vi "SubPanel_Oscilloscope_Block_Rev11_v2.vi"(2 "error input":errorcluster, 3 "Oscilloscope Configuration Input Array":T2(array[cluster]) {"vertical coupling" items=["AC", "DC", "Ground"]}) -> (0 "error out":errorcluster, 1 "Oscilloscope Configuration Output Array":T2(array[cluster]) {"vertical coupling" items=["AC", "DC", "Ground"]})   [LabVIEW 2019]
uses:
  Controls/OscilloscopeBlockControl.ctl
  <instrlib>/niScope/Controls/niScope vertical coupling.ctl
  <instrlib>/niScope/Configure/Trigger/niScope Configure Trigger Software.vi
panel:
  out "Oscilloscope Configuration Array Indicator":T2(array[cluster]) {"vertical coupling" items=["AC", "DC", "Ground"]}
  in  "Remove An Oscilloscope":bool
  in  "Oscilloscope Configuration Input Array":T3(array[cluster]) {"vertical coupling" items=["AC", "DC", "Ground"]}
  out "Horizontal:Actual Record Length":i32
  out "Configuration Errors":errorcluster
  in  "Oscilloscope Block Parameters":T4={"Oscilloscope"="", "channel names list"="", "vertical range"=10.0, "vertical coupling"=1, "Channel 0 50 ohms?"=FALSE, "50 ohm vertical range (V)"=10.0, "min record length"=1000, "min sample rate"=20000000.0} {"min sample rate" format="%^.2e"; "vertical coupling" items=["AC", "DC", "Ground"]}
  in  "EXIT SubVI":bool
  in  "Apply Configuration":bool
  # "Instructions\n\nSelect Oscilloscope Resource under \"Oscilloscope\"\n\nin a comma separate form (line 1, line 2, ...) type in the channel names of the device. \nIMPORTANT NOTE: \"line 1, line 2, ...\" will correspond to \"channel 0, channel 1, ...\" for each oscilloscope resource\n\nset the vertical range (no greater than 30)\n\nset the vertical coupling (dc) \n\nSet the channel 0 to 50 ohm impedance if you have something that requires 50 ohms to measure\n\nset 50 ohm vertical range if you have selected channel 0 50 ohms as true (ensure that it is no greater than 10\n\nmin record length (1000)\n\nmin sample rate (20e6) if you want a higher resolution, you increase the sample rate\n\npress apply configuration \n\nreview the instrument array above echoing your parameters created\n\nif you wish to remove a resource, select the oscilloscope resource in the \"oscillscope\" drop down\n\npress \"remove an oscilloscope\"\n\nonce fully configured, press \"EXIT\""
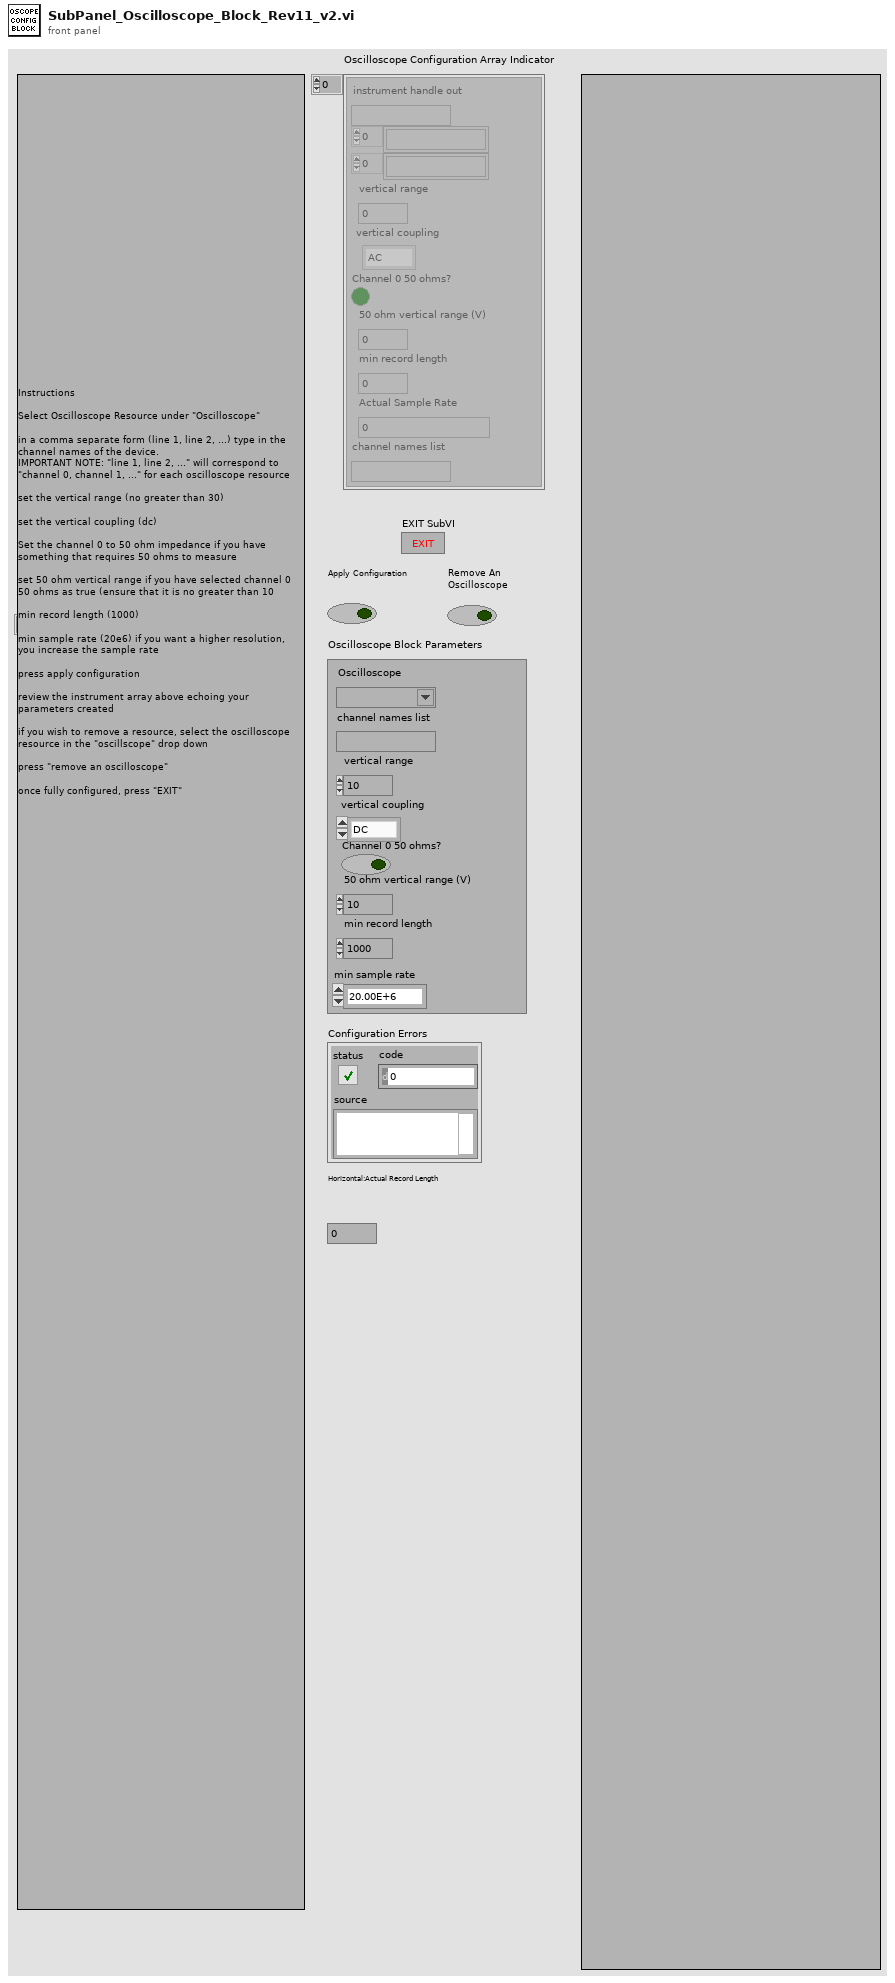
[diagram p1: front panel]
types:
  T1 = typedef "niScope vertical coupling.ctl" = i32
  T2 = cluster{"instrument handle out":refnum<k15>, string[], string[], "vertical range":dbl, "vertical coupling":T1, "Channel 0 50 ohms?":bool, "50 ohm vertical range (V)":dbl, "min record length":i32, "Actual Sample Rate":dbl, "channel names list":string}[]
  T3 = cluster{"instrument handle out":refnum<k15>, "channel numbers array":string[], "channel names array":string[], "vertical range":dbl, "vertical coupling":T1, "Channel 0 50 ohms?":bool, "50 ohm vertical range (V)":dbl, "min record length":i32, "Actual Sample Rate":dbl}[]
  T4 = typedef "OscilloscopeBlockControl.ctl" = cluster{"Oscilloscope":refnum<k15>, "channel names list":string, "vertical range":dbl, "vertical coupling":T1, "Channel 0 50 ohms?":bool, "50 ohm vertical range (V)":dbl, "min record length":i32, "min sample rate":dbl}
  T5 = cluster{"instrument handle out":refnum<k15>, string[], string[], "vertical range":dbl, "vertical coupling":T1, "Channel 0 50 ohms?":bool, "50 ohm vertical range (V)":dbl, "min record length":i32, "Actual Sample Rate":dbl, string}
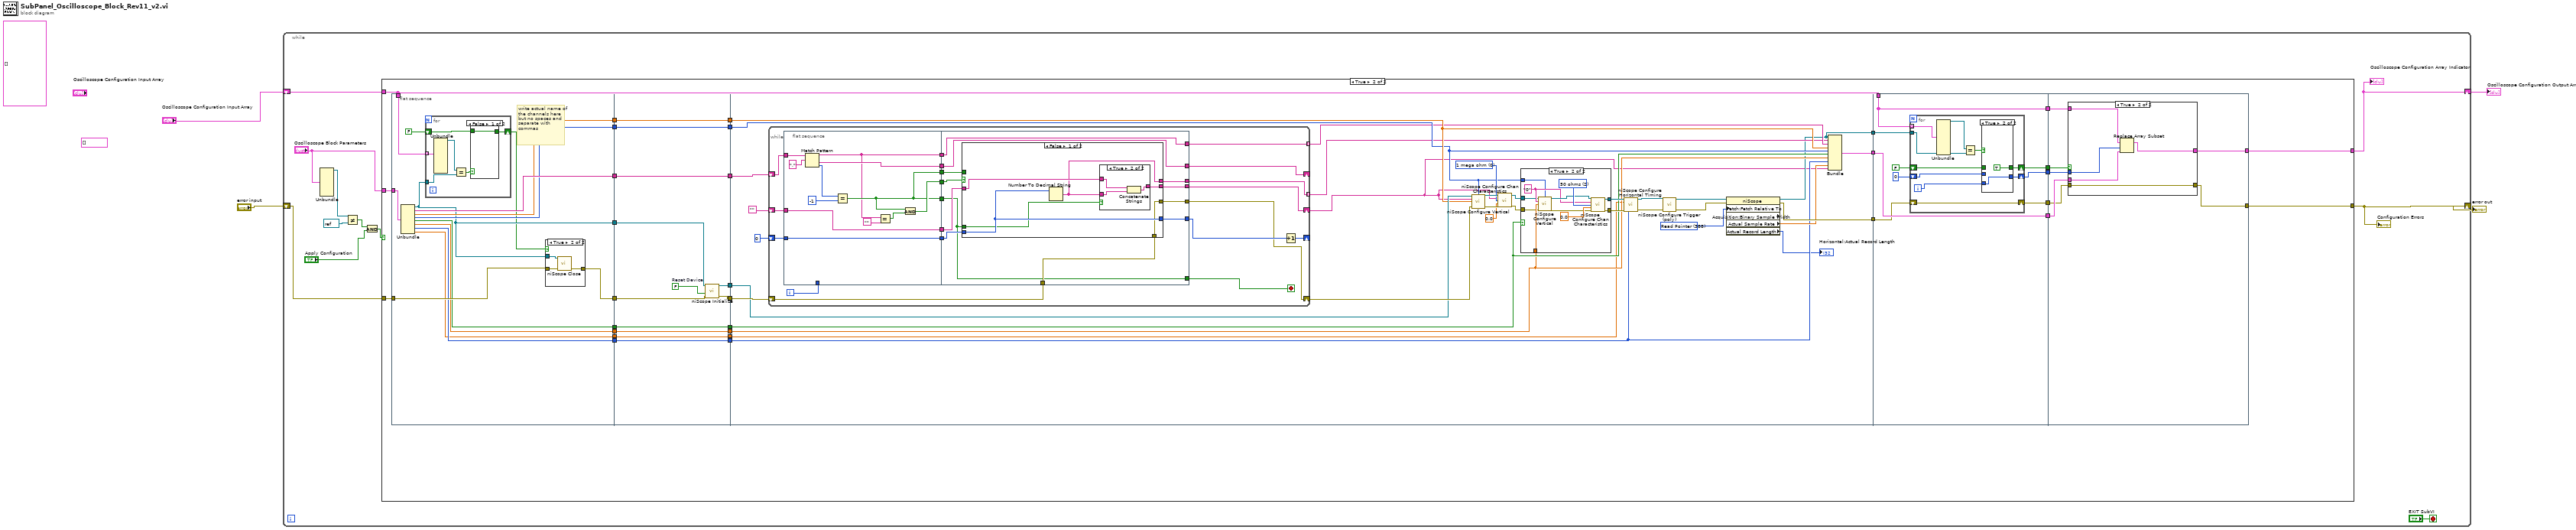
[diagram p0: block diagram]
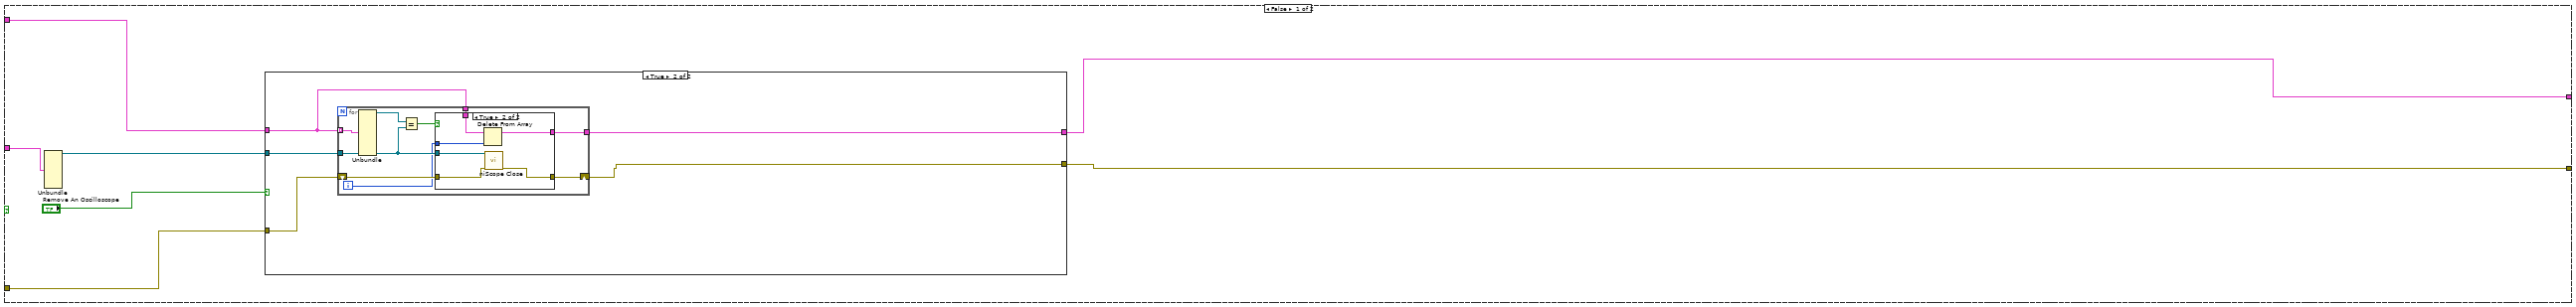
[diagram p2: hidden frame]
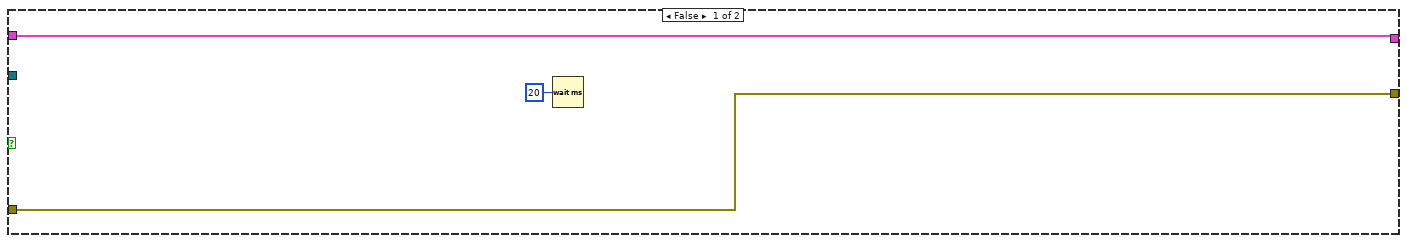
[diagram p3: hidden frame]
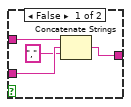
[diagram p7: hidden frame]
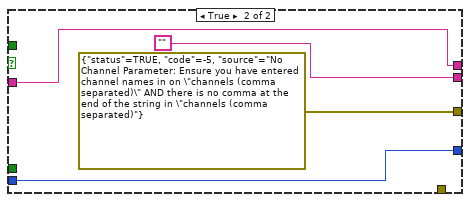
[diagram p8: hidden frame]
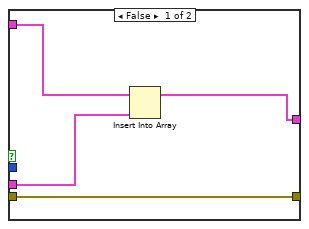
[diagram p11: hidden frame]
diagram:
  (unwired) T2 []
  (unwired) T3 [] ("Oscilloscope Configuration Input Array")
  n1 = while {
    shift-right: [w15] -> w4
    shift-left: "error input" -> [w13]
    shift-right: [w5] -> w1
    shift-left: "Oscilloscope Configuration Input Array" -> [w12]
    stop <- "EXIT SubVI" stop-if-true
    n2 = Unbundle("Oscilloscope Block Parameters") -> ("Oscilloscope"=w9:refnum<k15>)  [unwired: 7 out]
    n3 = Not Equal?(x=w9, y=refnum<k15> refnum ("resource name")) -> (x != y?=w8:bool)
    n4 = And(x=w8, y="Apply Configuration") -> (x .and. y?=w6:bool)
    n5 = case shown="True" w6 {
      tunnel: w13 -> [w19 w78]
      tunnel: [w18 w73] -> w15
      tunnel: [w16 w72] -> w5
      tunnel: w12 -> [w17 w48]
      tunnel: "Oscilloscope Block Parameters" -> [w22 w49]
      frame False {
        n6 = Unbundle(w22) -> ("Oscilloscope"=w20:refnum<k15>)  [unwired: 7 out]
        n7 = case shown="True" "Remove An Oscilloscope" {
          tunnel: w20 -> [_ w30]
          tunnel: w19 -> [w25 w29]
          tunnel: [w25 w26] -> w18
          tunnel: w17 -> [w23 w28]
          tunnel: [w23 w27] -> w16
          frame False {
            n8 = Wait (ms)(milliseconds to wait=u32 20) -> ()  [unwired: 1 out]
          }
          frame True {
            n9 = for {
              tunnel: w28 -> [w39] mode=indexing
              tunnel: w30 -> [w36]
              shift-right: [w34] -> w26
              shift-left: w29 -> [w35]
              tunnel: w28 -> [w33]
              tunnel: [w31] -> w27
              i -> [w32]
              n10 = Unbundle(w39) -> ("instrument handle out"=w38:refnum<k15>)  [unwired: 9 out]
              n11 = Equal?(x=w38, y=w36) -> (x = y?=w37:bool)
              n12 = case shown="True" w37 {
                tunnel: w36 -> [_ w47]
                tunnel: w35 -> [w41 w46]
                tunnel: [w41 w45] -> w34
                tunnel: w33 -> [w40 w44]
                tunnel: w32 -> [_ w43]
                tunnel: [w40 w42] -> w31
                frame False {
                }
                frame True {
                  n13 = Delete From Array(array=w44, index=w43) -> (array with subset deleted=w42:T2)  [unwired: 1 in, 1 out]
                  n14 = call <instrlib>:"niScope Close.vi"("instrument handle"=w47, "error in"=w46) -> ("error out"=w45:errorcluster)  [unwired: 13 in]
                }
              }
            }
          }
        }
      }
      frame True {
        n15 = flat-sequence {
          tunnel: w78 -> [w92]
          tunnel: [w91] -> w74
          tunnel: [w81] -> w71
          tunnel: [w90] -> w70
          tunnel: [w89] -> w68
          tunnel: [w88] -> w66
          tunnel: [w87] -> w64
          tunnel: [w86] -> w62
          tunnel: [w85] -> w60
          tunnel: [w84] -> w58
          tunnel: w49 -> [w83]
          tunnel: w48 -> [w82]
          tunnel: [w112] -> w77
          tunnel: [w114] -> w76
          tunnel: [w113] -> w75
          tunnel: w74 -> [w115]
          tunnel: w71 -> [w111]
          tunnel: w70 -> [w112]
          tunnel: [w110] -> w69
          tunnel: w68 -> [w110]
          tunnel: [w109] -> w67
          tunnel: w66 -> [w109]
          tunnel: [w108] -> w65
          tunnel: w64 -> [w108]
          tunnel: [w107] -> w63
          tunnel: w62 -> [w107]
          tunnel: [w106] -> w61
          tunnel: w60 -> [w106]
          tunnel: [w105] -> w59
          tunnel: w58 -> [w105]
          tunnel: w75 -> [w131]
          tunnel: w76 -> [w134]
          tunnel: w77 -> [w120]
          tunnel: w69 -> [w130]
          tunnel: w67 -> [w129]
          tunnel: w65 -> [w128]
          tunnel: w63 -> [w127]
          tunnel: w61 -> [w126]
          tunnel: w59 -> [w125]
          tunnel: [w137] -> w57
          tunnel: [w132] -> w56
          tunnel: [w121] -> w55
          tunnel: w57 -> [w225]
          tunnel: w56 -> [w232]
          tunnel: w55 -> [w231]
          tunnel: w48 -> [w227]
          tunnel: [w224] -> w54
          tunnel: [w232] -> w53
          tunnel: [w228] -> w52
          tunnel: [w227] -> w51
          tunnel: [w226] -> w50
          tunnel: [w250] -> w72
          tunnel: [w247] -> w73
          tunnel: w54 -> [w248]
          tunnel: w53 -> [w249]
          tunnel: w52 -> [w253]
          tunnel: w51 -> [w252]
          tunnel: w50 -> [w251]
          frame #0 {
            # "write actual name of the channels here but no spaces and separate with commas"
            n16 = Unbundle(w83) -> ("Oscilloscope"=w81:refnum<k15>, "channel names list"=w90:string, "vertical range"=w89:dbl, "vertical coupling"=w88:T1, "Channel 0 50 ohms?"=w87:bool, "50 ohm vertical range (V)"=w86:dbl, "min record length"=w85:i32, "min sample rate"=w84:dbl)
            n17 = for {
              tunnel: w82 -> [w98] mode=indexing
              tunnel: w81 -> [w97]
              shift-right: [w94] -> w79
              shift-left: FALSE -> [w93]
              n18 = Unbundle(w98) -> ("instrument handle out"=w96:refnum<k15>)  [unwired: 9 out]
              n19 = Equal?(x=w96, y=w97) -> (x = y?=w95:bool)
              n20 = case shown="False" w95 {
                selector: w95 -> [_ w100]
                tunnel: [w99 w100] -> w94
                tunnel: w93 -> [w99 _]
                frame False {
                }
                frame True {
                }
              }
            }
            n21 = case shown="True" w79 {
              tunnel: w81 -> [_ w102]
              tunnel: w92 -> [w101 w104]
              tunnel: [w101 w103] -> w91
              frame False {
              }
              frame True {
                n22 = call <instrlib>:"niScope Close.vi"("instrument handle"=w102, "error in"=w104) -> ("error out"=w103:errorcluster)  [unwired: 13 in]
              }
            }
          }
          frame #1 {
            w116 = FALSE  # Reset Device
            n23 = call <instrlib>:"niScope Initialize.vi"("resource name"=w111, "reset device"=w116, "error in"=w115) -> ("instrument handle"=w113:refnum<k15>, "error out"=w114:errorcluster)  [unwired: 11 in]
          }
          frame #2 {
            w140 = 388 items=["Start"=482, "Trigger"=483, "Pretrigger"=477, "Now"=481, "Read Pointer"=388] ("Fetch:Fetch Relative To")
            w146 = u32 0 items=["1 mega ohm"=0, "50 ohms"=2] ("input impedance")
            n24 = while {
              shift-right: [w168] -> _
              shift-left: w120 -> [w169]
              shift-right: [w156] -> _
              shift-left: 0 -> [w161]
              shift-right: [w153] -> w119
              shift-left: "" -> [w159]
              tunnel: [w152] -> w124 mode=indexing
              shift-right: [w154] -> w149
              shift-left: w134 -> [w158]
              tunnel: [w150] -> w123 mode=indexing
              i -> [w167]
              stop <- w166 stop-if-true
              n25 = flat-sequence {
                tunnel: w169 -> [w179]
                tunnel: w167 -> [_]
                tunnel: [w177] -> w165
                tunnel: [w171] -> w164
                tunnel: [w172] -> w163
                tunnel: [w176] -> w162
                tunnel: w161 -> [w176]
                tunnel: [w175] -> w160
                tunnel: w159 -> [w175]
                tunnel: [w171] -> w155
                tunnel: [w170] -> w151
                tunnel: w165 -> [w193]
                tunnel: w164 -> [w184]
                tunnel: w163 -> [w192]
                tunnel: w162 -> [w190]
                tunnel: w160 -> [w189]
                tunnel: w158 -> [w188]
                tunnel: [w193] -> w168
                tunnel: [w184] -> w166
                tunnel: [w191] -> w153
                tunnel: [w187] -> w154
                tunnel: [w186] -> w157
                tunnel: w155 -> [w185]
                tunnel: [w183] -> w152
                tunnel: w151 -> [w183]
                tunnel: [w182] -> w150
                frame #0 {
                  n26 = Match Pattern(string=w179, regular expression=",") -> (before substring=w170:string, after substring=w177:string, offset past match=w181:i32)  [unwired: 1 in, 1 out]
                  n27 = Equal?(x=w181, y=-1) -> (x = y?=w171:bool)
                  n28 = Equal?(x=w170, y="") -> (x = y?=w173:bool)
                  n29 = And(x=w171, y=w173) -> (x .and. y?=w172:bool)
                }
                frame #1 {
                  n30 = case shown="False" w192 {
                    tunnel: [w195 ""] -> w191
                    tunnel: w190 -> [w199 w209]
                    tunnel: w189 -> [w197 w207]
                    tunnel: [w199 w209] -> w186
                    tunnel: w188 -> [w198 _]
                    tunnel: [w198 errorcluster {"status"=TRUE, "code"=-5, "source"="No Channel Parameter: Ensure you have entered channel names in on \"channels (comma separated)\" AND there is no comma at the end of the string in \"channels (comma separated)"} ("error out")] -> w187
                    tunnel: w185 -> [_ _]
                    tunnel: w184 -> [w196 _]
                    tunnel: [w194 w207] -> w182
                    frame False {
                      n31 = Number To Decimal String(number=w199) -> (decimal integer string=w194:string)  [unwired: 1 in]
                      n32 = case shown="True" w196 {
                        tunnel: w197 -> [w203 w206]
                        tunnel: w194 -> [w202 w205]
                        tunnel: [w200 w204] -> w195
                        frame False {
                          n33 = Concatenate Strings(w203, w202, "," ("string")) -> (w200:string)
                        }
                        frame True {
                          n34 = Concatenate Strings(w206, w205) -> (w204:string)
                        }
                      }
                    }
                    frame True {
                    }
                  }
                }
              }
              n35 = Increment(x=w157) -> (x+1=w156:i32)
            }
            n36 = call <instrlib>:"niScope Configure Vertical.vi"("instrument handle"=w131, "vertical coupling"=w129, "channels"=w119, "vertical range"=w130, "error in"=w149) -> ("instrument handle out"=w148:refnum<k15>, "error out"=w147:errorcluster)  [unwired: 9 in]
            n37 = call <instrlib>:"niScope Configure Chan Characteristics.vi"("instrument handle"=w148, "channels"=w119, "input impedance"=w146, "maximum input frequency"=0.0, "error in"=w147) -> ("instrument handle out"=w144:refnum<k15>, "error out"=w143:errorcluster)  [unwired: 9 in]
            n38 = case shown="True" w128 {
              tunnel: [w212 w223] -> w139
              tunnel: [w211 w222] -> w138
              tunnel: w127 -> [_ w216]
              tunnel: w144 -> [w212 w215]
              tunnel: w143 -> [w211 w214]
              tunnel: w129 -> [_ w213]
              frame False {
              }
              frame True {
                w220 = u32 2 items=["1 mega ohm"=0, "50 ohms"=2] ("input impedance")
                w217 = "0" ("channels")
                n39 = call <instrlib>:"niScope Configure Vertical.vi"("instrument handle"=w215, "vertical coupling"=w213, "channels"=w217, "vertical range"=w216, "error in"=w214) -> ("instrument handle out"=w219:refnum<k15>, "error out"=w218:errorcluster)  [unwired: 9 in]
                n40 = call <instrlib>:"niScope Configure Chan Characteristics.vi"("instrument handle"=w219, "channels"=w217, "input impedance"=w220, "maximum input frequency"=0.0, "error in"=w218) -> ("instrument handle out"=w223:refnum<k15>, "error out"=w222:errorcluster)  [unwired: 9 in]
              }
            }
            n41 = call <instrlib>:"niScope Configure Horizontal Timing.vi"("instrument handle"=w139, "min sample rate"=w125, "error in"=w138, "min record length"=w126) -> ("instrument handle out"=w142:refnum<k15>, "error out"=w141:errorcluster)  [unwired: 10 in]
            n42 = call-poly <instrlib>:"niScope Configure Trigger (poly).vi"("instrument handle"=w142, "error in"=w141) -> ("instrument handle out"=w118:refnum<k15>, "error out"=w117:errorcluster)  [unwired: 12 in]
            n43 = property class="niScope" props=["Fetch:Fetch Relative To", "Acquisition:Binary Sample Width", "Actual Sample Rate", "Actual Record Length"](reference=w118, error in=w117, "Fetch:Fetch Relative To"=w140) -> (reference out=w121:refnum<k15>, error out=w137:errorcluster, "Actual Sample Rate"=w133:dbl, "Actual Record Length"=→"Horizontal:Actual Record Length":i32)  [unwired: 1 out]
            n44 = Bundle("instrument handle out"=w121, w123, w124, "vertical range"=w130, "vertical coupling"=w129, "Channel 0 50 ohms?"=w128, "50 ohm vertical range (V)"=w127, "min record length"=w126, "Actual Sample Rate"=w133, w119) -> (w132:T5)  [unwired: 1 in]
          }
          frame #3 {
            n45 = for {
              tunnel: w227 -> [w242] mode=indexing
              tunnel: w231 -> [w240]
              shift-right: [w237] -> w228
              shift-left: FALSE -> [w238]
              shift-right: [w235] -> w226
              shift-left: 0 -> [w236]
              shift-right: [w233] -> w224
              shift-left: w225 -> [w233]
              i -> [w234]
              n46 = Unbundle(w242) -> ("instrument handle out"=w241:refnum<k15>)  [unwired: 9 out]
              n47 = Equal?(x=w241, y=w240) -> (x = y?=w239:bool)
              n48 = case shown="True" w239 {
                tunnel: w238 -> [w244 _]
                tunnel: [w244 TRUE] -> w237
                tunnel: w236 -> [w243 _]
                tunnel: [w243 w245] -> w235
                tunnel: w234 -> [_ w245]
                frame False {
                }
                frame True {
                }
              }
            }
          }
          frame #4 {
            n49 = case shown="True" w253 {
              tunnel: w252 -> [w257 w262]
              tunnel: w249 -> [w256 w261]
              tunnel: w251 -> [_ w260]
              tunnel: [w255 w259] -> w250
              tunnel: [w254 w258] -> w247
              tunnel: w248 -> [w254 w258]
              frame False {
                n50 = Insert Into Array(array=w257, new element=w256) -> (w255:T2)  [unwired: 1 in]
              }
              frame True {
                n51 = Replace Array Subset(array=w262, new element=w261, index=w260) -> (w259:T2)
              }
            }
          }
        }
      }
    }
    "Configuration Errors" <- w15
    "Oscilloscope Configuration Array Indicator" <- w5
  }
  "error out" <- w4
  "Oscilloscope Configuration Output Array" <- w1
